vi "Write COE file.vi"() -> ()   [LabVIEW 2016]
uses:
  Waveform parameters.ctl
panel:
  out "Waveform parameters out":T1={"Start magnitude"=0.0, "Magnitude increment"=0.0, "Number of pulses"=0, "Baseline length"=0, "Ramp length"=0, "Top  length"=0, "Threshold "=3000}
  in  "Waveform parameters":T1={"Start magnitude"=1000.0, "Magnitude increment"=1000.0, "Number of pulses"=8, "Baseline length"=480, "Ramp length"=32, "Top  length"=480, "Threshold "=3000}
  in  "File Path Control":path=path "D:/github/fp/Simulation/BRAM.coe"
  out "spreadsheet string":string
  out "Step length":u32=2048
  out "Waveform length":u32
  out "Waveform Graph":dbl[](graph)
  in  "Baseline start":u16=128
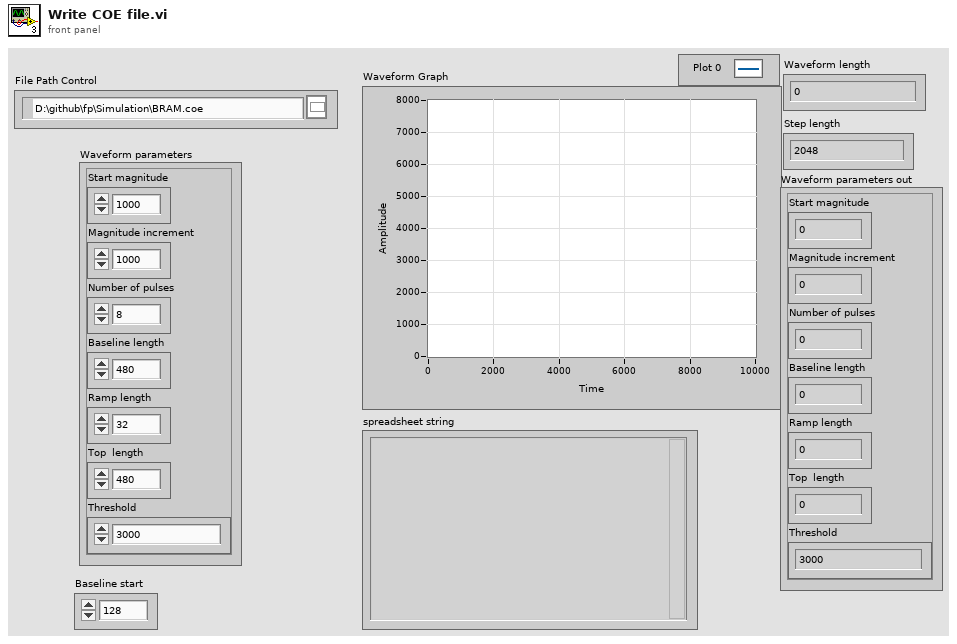
[diagram p1: front panel]
types:
  T1 = typedef "Waveform parameters.ctl" = cluster{"Start magnitude":dbl, "Magnitude increment":dbl, "Number of pulses":i32, "Baseline length":i32, "Ramp length":i32, "Top  length":i32, "Threshold ":i32}
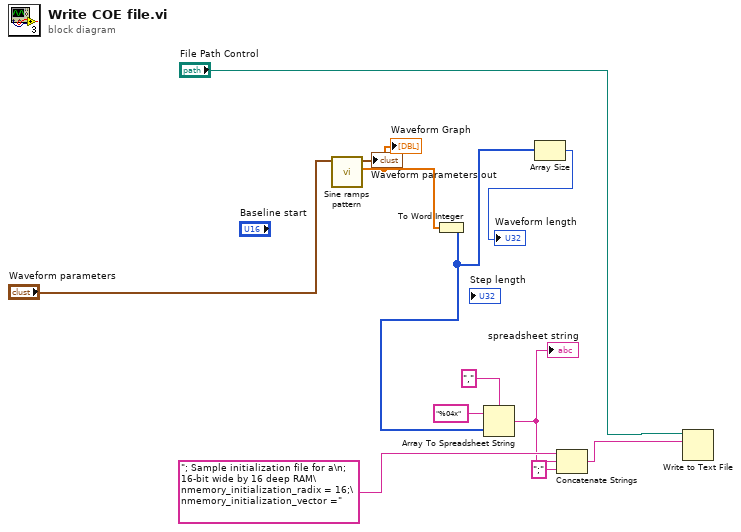
[diagram p0: block diagram]
diagram:
  n1 = call "Sine ramps pattern.vi"("Waveform parameters 2"="Waveform parameters") -> ("Waveform"=w4:dbl[], "Waveform parameters out"=→"Waveform parameters out":T1)  [unwired: 8 in]
  "Waveform Graph" <- w4
  n2 = To Word Integer(number=w4) -> (16bit integer=w2:i16[])
  n3 = Array To Spreadsheet String(delimiter (Tab)=",", array=w2, 3:"%04x" ("format string")) -> (spreadsheet string=w8:string)
  "spreadsheet string" <- w8
  n4 = Array Size(array=w2) -> (size(s)=→"Waveform length":i32)
  n5 = Concatenate Strings("; Sample initialization file for a\n; 16-bit wide by 16 deep RAM\nmemory_initialization_radix = 16;\nmemory_initialization_vector =" ("text"), w8, ";" ("string")) -> (w7:string)
  n6 = Write to Text File(file (use dialog)="File Path Control", text=w7) -> ()  [unwired: 2 in, 3 out]
